vi "LvIRKit_SUB_Messages_GET.vi"(8 "error in (no error)":errorcluster, 11 "IRKit IP address":string) -> (0 "error out":errorcluster, 2 "Message":string)   [LabVIEW 2014]
uses:
  <vilib>/httpClient/LabVIEWHTTPClient.lvlib
panel:
  # "LvIRKit:: Message GET"
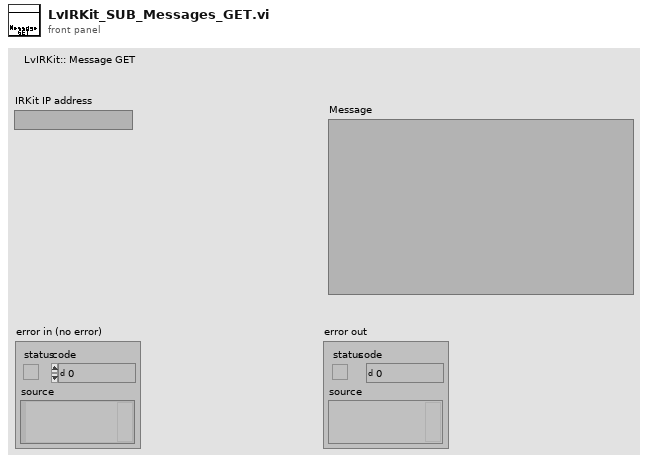
[diagram p1: front panel]
types:
  T1 = typedef "LabVIEWHTTPClient.lvlib/ClientHandle.ctl" = refnum<k1>
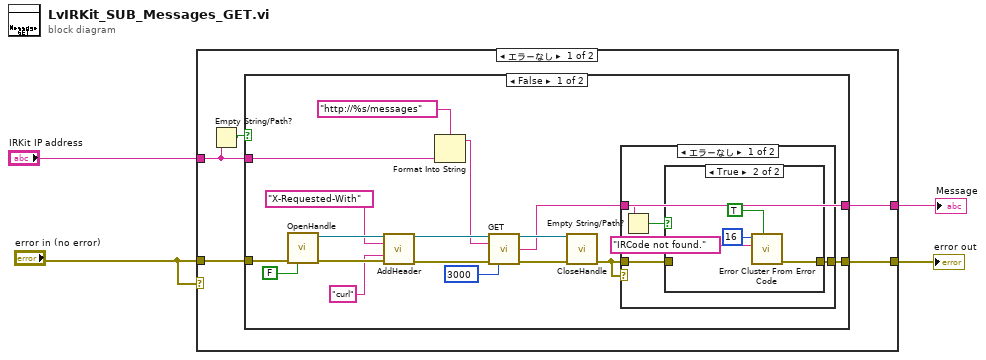
[diagram p0: block diagram]
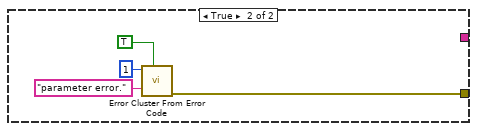
[diagram p4: hidden frame]
diagram:
  n1 = case shown="エラーなし" "error in (no error)" {
    tunnel: [w9 w41] -> w4
    tunnel: "error in (no error)" -> [w8 w41]
    tunnel: [w7 _] -> w3
    tunnel: "IRKit IP address" -> [w5 _]
    frame No Error {
      n2 = Empty String/Path?(string/path=w5) -> (empty?=w6:bool)
      n3 = case shown="FALSE" w6 {
        tunnel: [w11 w40] -> w9
        tunnel: w8 -> [w15 _]
        tunnel: [w12 _] -> w7
        tunnel: w5 -> [w14 _]
        frame False {
          n4 = call <vilib>:"OpenHandle.vi"("error in (no error)"=w15, "verify server(true)"=FALSE) -> ("client handle out"=w23:T1, "error out"=w26:errorcluster)  [unwired: 12 in]
          n5 = call <vilib>:"AddHeader.vi"("client handle"=w23, "header"="X-Requested-With" ("url"), "value"="curl" ("url"), "error in (no error)"=w26) -> ("client handle out"=w24:T1, "error out"=w25:errorcluster)  [unwired: 10 in]
          n6 = Format Into String(format string="http://%s/messages", w14) -> (resulting string=w19:string)  [unwired: 2 in, 1 out]
          n7 = call <vilib>:"GET.vi"("client handle"=w24, "url"=w19, "error in (no error)"=w25, "timeout (10000)"=3000) -> ("client handle out"=w17:T1, "body"=w12:string, "error out"=w18:errorcluster)  [unwired: 8 in, 1 out]
          n8 = call <vilib>:"CloseHandle.vi"("client handle"=w17, "error in (no error)"=w18) -> ("error out"=w10:errorcluster)  [unwired: 13 in]
          n9 = case shown="エラーなし" w10 {
            tunnel: w12 -> [w30 _]
            tunnel: w10 -> [w28 w36]
            tunnel: [w27 w36] -> w11
            frame No Error {
              n10 = Empty String/Path?(string/path=w30) -> (empty?=w29:bool)
              n11 = case shown="TRUE" w29 {
                tunnel: w28 -> [w31 _]
                tunnel: [w31 w35] -> w27
                frame False {
                }
                frame True {
                  n12 = call <vilib>:"Error Cluster From Error Code.vi"("show call chain? (False)"=TRUE, "error message (\"\")"="IRCode not found." ("error message (\"\")"), "error code (0)"=16) -> ("error out"=w35:errorcluster)  [unwired: 6 in]
                }
              }
            }
            frame Error {
            }
          }
        }
        frame True {
          n13 = call <vilib>:"Error Cluster From Error Code.vi"("show call chain? (False)"=TRUE, "error message (\"\")"="parameter error." ("error message (\"\")"), "error code (0)"=1) -> ("error out"=w40:errorcluster)  [unwired: 6 in]
        }
      }
    }
    frame Error {
    }
  }
  "error out" <- w4
  "Message" <- w3
